vi "Test.vi"(8 "Voie physique DAQmx":tag="sHIT/ai0") -> (0 "waveform en sortie":waveform(dbl))   [LabVIEW 2013]
uses:
  <vilib>/DAQmx/read.llb/DAQmx Read (Analog Wfm 1Chan NSamp).vi
  <vilib>/DAQmx/miscellaneous.llb/DAQmx Fill In Error Info.vi
  <vilib>/express/express analysis/Spectral/Block/exnSpectralBlock spectral measurements PSD poly.vi
  <vilib>/express/express analysis/Spectral/Block/exnSpectralBlock spectral measurements PSD WFM.vi
  <vilib>/express/express analysis/Spectral/XNode/ExpressSpectralMeasurementsBlockNode.xnode
panel:
  in  "Signal de Reference":T1(ring)
  in  "Offset":dbl
  in  "Amplitude":dbl
  in  "Phase":dbl
  in  "Frequence 2":dbl
  in  "Statistiques":bool
  out "Moyenne":dbl
  out "Valeur eff":dbl
  out "Frequence":dbl
  in  "FFT":bool
  in  "Fenetre d'affichage (s)":dbl step=0.001
  out "Signal":waveform(dbl)[](graph)
  out "FFT":cluster{"f0":dbl, "df":dbl, "magnitude":dbl[]}(graph)
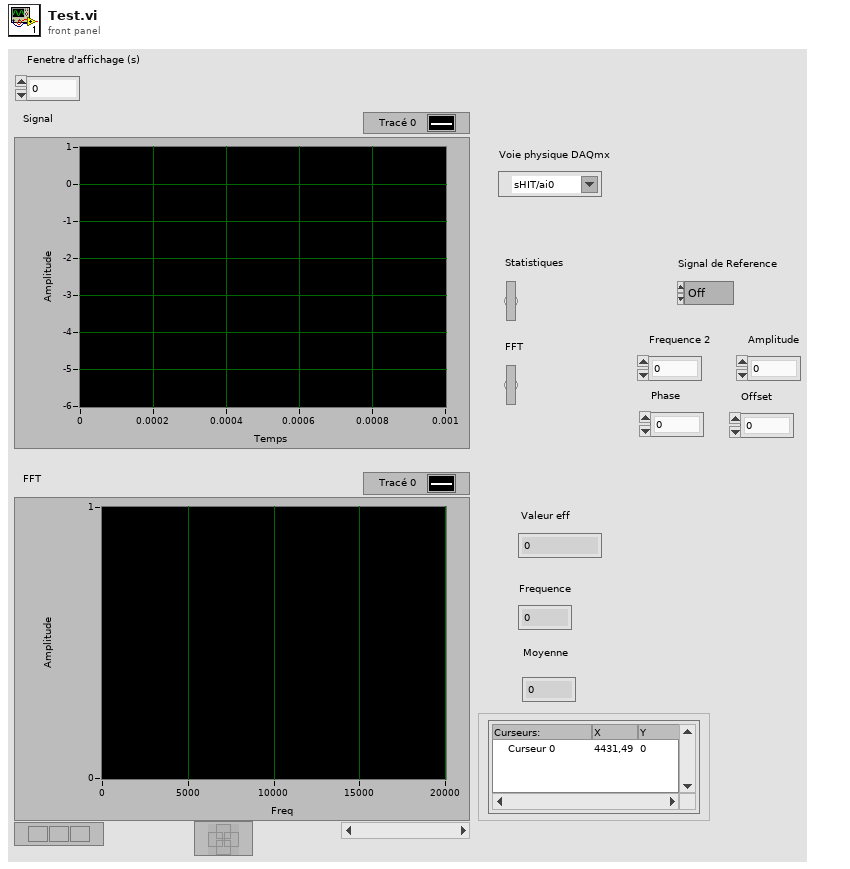
[diagram p1: front panel]
types:
  T1 = enum16{"Off", "Sinus", "Carre", "Triangle", "Scie"}
  T2 = enum16{"Off", "Sinus", "Carre", "Triangle", "Scie", ""}
  T3 = cluster{"averaging mode":u16, "weighting mode":u16, "number of averages":u32}
  T4 = cluster{"dB On (F)":bool, "unwrap phase (F)":bool, "convert to degree (F)":bool}
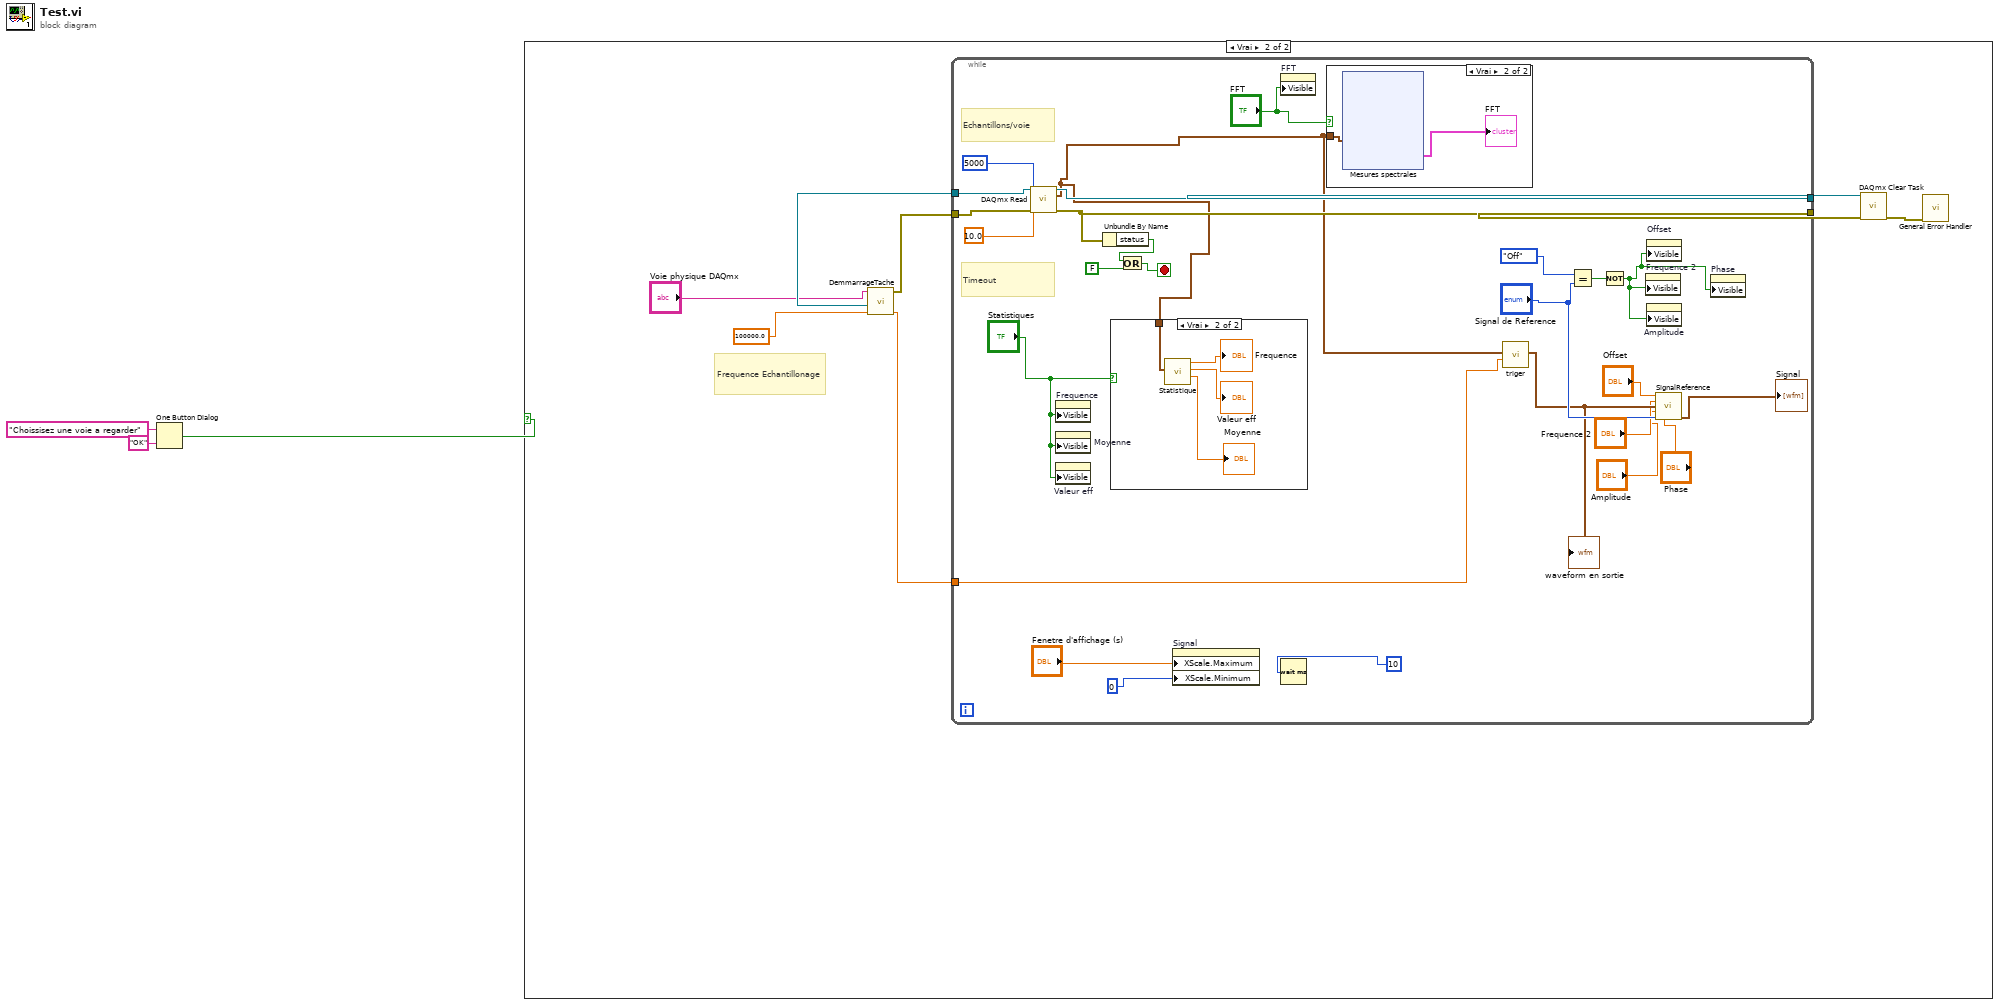
[diagram p0: block diagram]
diagram:
  n1 = One Button Dialog(message="Choissisez une voie a regarder", button name ("OK")="OK" ("nom du bouton (\"OK\")")) -> (true=w1:bool)
  n2 = case shown="Vrai" w1 {
    frame False {
    }
    frame True {
      # "Frequence Echantillonage"
      n3 = call "DemmarrageTache.vi"("frequence echantillonage"=100000.0, "Voie physique DAQmx"="Voie physique DAQmx") -> ("frequence echantillonage 2"=w5:dbl, "task out"=w6:refnum<k21>, "error out"=w7:errorcluster)  [unwired: 6 in]
      n4 = while {
        tunnel: w6 -> [w37]
        tunnel: w7 -> [w36]
        tunnel: [w34] -> w11
        tunnel: [w30] -> w10
        tunnel: w5 -> [w22]
        stop <- w33 stop-if-true
        # "Echantillons/voie"
        # "Timeout"
        n5 = call-poly <vilib>:"DAQmx Read.vi"("task/channels in"=w37, "number of samples per channel"=5000, "timeout"=10.0, "error in"=w36) -> ("task out"=w34:refnum<k21>, "data"=w23:waveform(dbl), "error out"=w30:errorcluster)  [unwired: 9 in]
        n6 = property on="Frequence" class="NumNb (strict)"("Visible"="Statistiques") -> ()  [unwired: 2 in, 2 out]
        n7 = property on="Moyenne" class="NumNb (strict)"("Visible"="Statistiques") -> ()  [unwired: 2 in, 2 out]
        n8 = property on="Valeur eff" class="NumNb (strict)"("Visible"="Statistiques") -> ()  [unwired: 2 in, 2 out]
        n9 = Unbundle By Name(w30) -> ("status"=w31:bool)
        n10 = case shown="Vrai" "Statistiques" {
          tunnel: w23 -> [_ w41]
          frame False {
          }
          frame True {
            n11 = call "Statistique.vi"("Waveform"=w41) -> ("mean"=→"Moyenne":dbl, "Valeur efficace"=→"Valeur eff":dbl, "Fréquence"=→"Frequence":dbl)  [unwired: 8 in]
          }
        }
        n12 = Or(x=w31, y=FALSE) -> (x .or. y?=w33:bool)
        n13 = property on="Signal" class="GraphWF (strict)"("XScale.Maximum"="Fenetre d'affichage (s)", "XScale.Minimum"=0) -> ()  [unwired: 2 in, 2 out]
        n14 = property on="FFT" class="GraphWF (strict)"("Visible"="FFT") -> ()  [unwired: 2 in, 2 out]
        n15 = Wait (ms)(milliseconds to wait=10) -> ()  [unwired: 1 out]
        n16 = case shown="Vrai" "FFT" {
          tunnel: w23 -> [_ w42]
          frame False {
          }
          frame True {
            n17 = xnode "Mesures spectrales"("Signaux"=w42) -> ("DSP"=→"FFT":cluster{"f0":dbl, "df":dbl, "magnitude":dbl[]})  [unwired: 1 in, 1 out]
          }
        }
        n18 = call "triger.vi"("frequene echantillonage"=w22, "Signal"=w23) -> ("waveform en sortie"=w17:waveform(dbl))  [unwired: 9 in]
        "waveform en sortie" <- w17
        n19 = Equal?(x=T2."Off" ("Énum 2"), y="Signal de Reference") -> (x = y?=w20:bool)
        n20 = Not(x=w20) -> (.not. x?=w19:bool)
        n21 = property on="Frequence 2" class="NumNb (strict)"("Visible"=w19) -> ()  [unwired: 2 in, 2 out]
        n22 = property on="Offset" class="NumNb (strict)"("Visible"=w19) -> ()  [unwired: 2 in, 2 out]
        n23 = property on="Amplitude" class="NumNb (strict)"("Visible"=w19) -> ()  [unwired: 2 in, 2 out]
        n24 = call "SignalReference.vi"("Offset"="Offset", "Frequence 2"="Frequence 2", "waveform en sortie"=w17, "Amplitude"="Amplitude", "Signal de Reference"="Signal de Reference", "Phase"="Phase") -> ("Tableau"=→"Signal":waveform(dbl)[])  [unwired: 9 in]
        n25 = property on="Phase" class="NumNb (strict)"("Visible"=w19) -> ()  [unwired: 2 in, 2 out]
      }
      n26 = call <vilib>:"DAQmx Clear Task.vi"("task in"=w11, "error in"=w10) -> ("error out"=w9:errorcluster)  [unwired: 13 in]
      n27 = call <vilib>:"General Error Handler.vi"("error in (no error)"=w9) -> ()  [unwired: 10 in, 5 out]
    }
  }
